vi "Filter_CW.vi"() -> (5 "Plug in titles":string[](array[string]), 7 "Plug in values":string[](array[string]))   [LabVIEW 2010]
uses:
  Globals/Plug_in_data_global.vi
  Globals/Meas_global.vi
  <vilib>/Analysis/NI_AALBase.lvlib
  <vilib>/Analysis/3filter.llb/Butterworth Filter (DBL).vi
panel:
  out "Waveform Graph":dbl[][](graph)
  # "Run this VI to update the channel names"
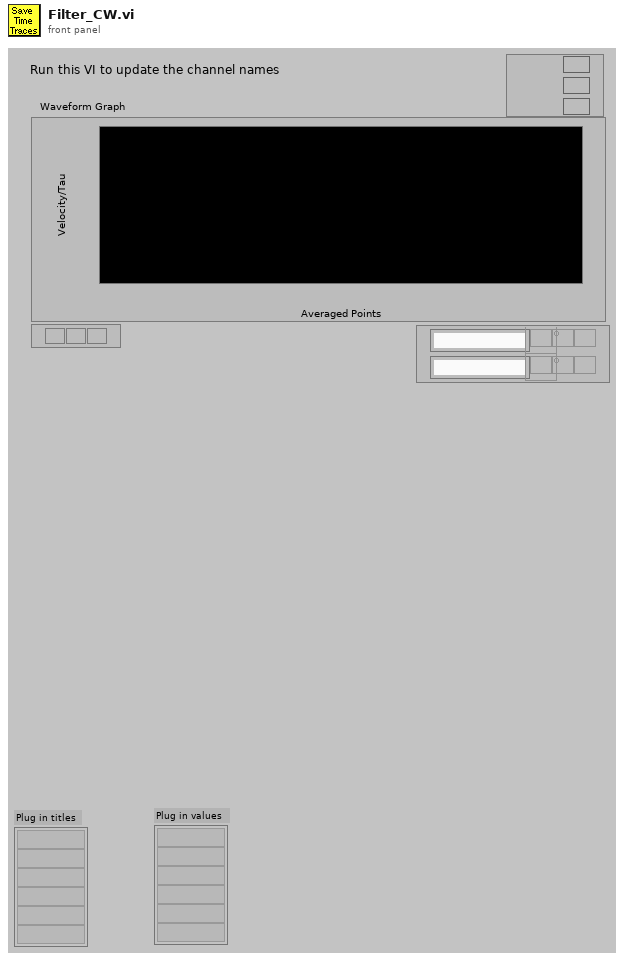
[diagram p1: front panel]
types:
  T1 = enum32{"Lowpass", "Highpass", "Bandpass", "Bandstop"}
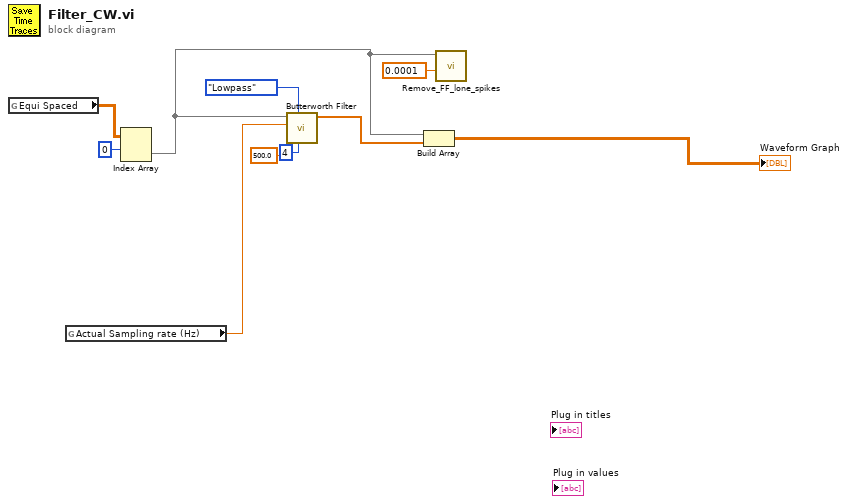
[diagram p0: block diagram]
diagram:
  n1 = global read "Plug_in_data_global.vi" "Equi Spaced"() -> (w10:dbl[][])
  n2 = global read "Meas_global.vi" "Actual Sampling rate (Hz)"() -> (w7:dbl)
  n3 = Index Array(array=w10, index (row)=0) -> (element=w3:dbl[])  [unwired: 1 in]
  n4 = call-poly <vilib>:"Butterworth Filter.vi"("order"=4, "filter type"=T1."Lowpass", "low cutoff freq: fl"=500.0 ("high cutoff freq: fh"), "sampling freq: fs"=w7, "X"=w3) -> ("Filtered X"=w6:dbl[])  [unwired: 2 in, 2 out]
  n5 = Build Array(w3, w6) -> (→"Waveform Graph":dbl[][])
  n6 = call "Remove_FF_lone_spikes.vi"("Bkgnd variance"=0.0001, "Time Trace"=w3) -> ()  [unwired: 2 in, 2 out]
